vi "Exec ssh-keygen.vi"(8 "error in (no error)":errorcluster, 10 "arguments":string) -> (0 "error out":errorcluster)   [LabVIEW 2013, in "libssh2_integration_tests.lvlib" / "Server Fixture.lvclass"]
doc: "Execute ssh-keygen with specified arguments."
uses:
  Server Fixture.lvclass
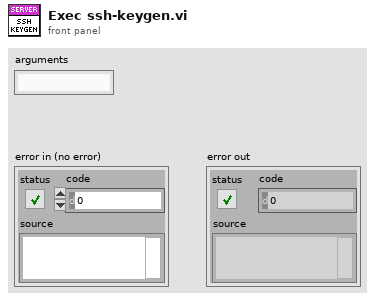
[diagram p1: front panel]
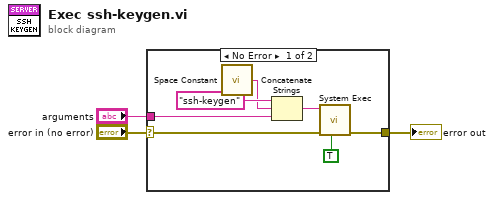
[diagram p0: block diagram]
diagram:
  n1 = case shown="No Error" "error in (no error)" {
    selector: "error in (no error)" -> [w4 w11]
    tunnel: "arguments" -> [w9 _]
    tunnel: [w5 w11] -> w2
    frame No Error {
      n2 = call <vilib>:"Space Constant.vi"() -> ("String"=w7:string)
      n3 = Concatenate Strings("ssh-keygen" ("executable"), w7, w9) -> (w6:string)
      n4 = call <vilib>:"System Exec.vi"("run minimized? (F)"=TRUE, "error in (no error)"=w4, "command line"=w6) -> ("error out"=w5:errorcluster)  [unwired: 5 in, 3 out]
    }
    frame Error {
    }
  }
  "error out" <- w2
